vi "subLoadConfigurationPage.vi"(9 "Parameters":string, 11 "Interface in":refnum<class>) -> (0 "error out":errorcluster, 3 "References":T1)   [LabVIEW 2020, in "DependencyInspector.lvlib"]
uses:
  DependencyInspector.lvlib
  ExtensionInterfaces/IConfigurationPage/Event_Stop.ctl
  ExtensionInterfaces/IConfigurationPage/IConfigurationPage.lvclass
  ExtensionInterfaces/IConfigurationPage/Event_Parameters.ctl
  Private/subReferenceData.ctl
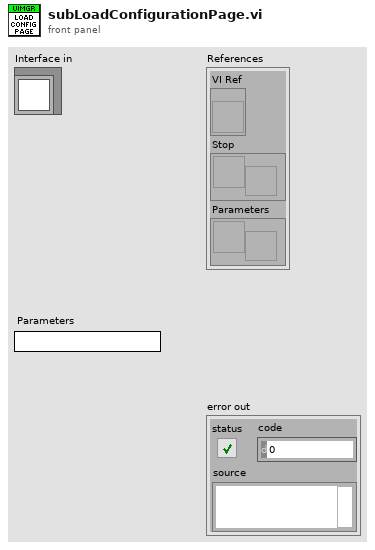
[diagram p1: front panel]
types:
  T1 = typedef "DependencyInspector.lvlib/subReferenceData.ctl" = cluster{"VI Ref":refnum<vi>, "Stop":refnum<user-event>, "Parameters":refnum<user-event>}
  T2 = typedef "ExtensionInterfaces.lvlib/IConfigurationPage.lvclass/Event_Parameters.ctl" = cluster{"Parameters":string}
  T3 = typedef "ExtensionInterfaces.lvlib/IConfigurationPage.lvclass/Event_Stop.ctl" = cluster{"Stop":bool}
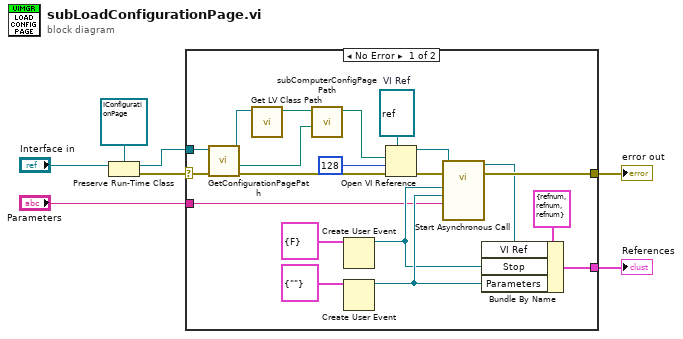
[diagram p0: block diagram]
diagram:
  n1 = Preserve Run-Time Class(object in="Interface in", 2:refnum<class "IConfigurationPage.lvclass"> refnum ("ExtensionInterfaces.lvlib:IConfigurationPage.lvclass")) -> (object out=w4:refnum<class "IConfigurationPage.lvclass">, error out=w6:errorcluster)  [unwired: 1 in]
  n2 = case shown="No Error" w6 {
    selector: w6 -> [w9 _]
    tunnel: w4 -> [w10 _]
    tunnel: [w20 _] -> w7
    tunnel: [w16 _] -> w2
    tunnel: "Parameters" -> [w8 _]
    frame No Error {
      w26 = refnum<vi> refnum  # VI Ref
      n3 = call-dynamic "GetConfigurationPagePath.vi"("error in (no error)"=w9, "IConfigurationPage in"=w10) -> ("error out"=w27:errorcluster, "Path"=w15:path, "IConfigurationPage out"=w13:refnum<class "IConfigurationPage.lvclass">)  [unwired: 7 in]
      n4 = call <vilib>:"Get LV Class Path.vi"("object"=w13) -> ("class path"=w12:path)  [unwired: 9 in, 1 out]
      n5 = call "subComputerConfigPagePath.vi"("Config page path"=w15, "Class path"=w12) -> ("Path out"=w14:path)  [unwired: 9 in]
      n6 = Create User Event(user event datatype=T3 {"Stop"=FALSE} ("Stop")) -> (user event=w18:refnum<user-event>)  [unwired: 1 in, 1 out]
      n7 = Create User Event(user event datatype=T2 {"Parameters"=""} ("Parameters")) -> (user event=w19:refnum<user-event>)  [unwired: 1 in, 1 out]
      n8 = Open VI Reference(type specifier VI Refnum (for type only)=w26, vi path=w14, options=128, error in (no error)=w27) -> (vi reference=w24:refnum<vi>, error out=w25:errorcluster)  [unwired: 2 in]
      n9 = call-by-ref "Start Asynchronous Call"(reference=w24, error in=w25, "Parameter defaults"=w8, "Parameters"=w19, "Stop"=w18) -> (reference out=w17:refnum<vi>, error out=w20:errorcluster)  [unwired: 9 in]
      n10 = Bundle By Name(cluster=T1 {"VI Ref"=refnum, "Stop"=refnum, "Parameters"=refnum} ("References"), "VI Ref"=w17, "Stop"=w18, "Parameters"=w19) -> (w16:T1)
    }
    frame Error {
    }
  }
  "References" <- w2
  "error out" <- w7
